vi "test.vi"() -> ()   [LabVIEW 2020, in "MSXML.lvlib"]
uses:
  Public/Type Definition/Attributes__slk_msxml.ctl
  Public/Type Definition/Attribute__slk_msxml.ctl
  MSXML.lvlib
  Public/MSXML Document/msxml document.lvclass
  Public/MSXML Node/msxml node.lvclass
panel:
  out "xml data":string
  in  "attributes":T1
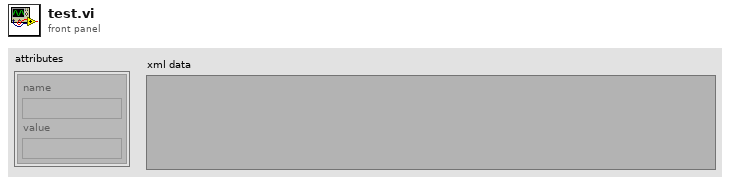
[diagram p1: front panel]
types:
  T1 = typedef "MSXML.lvlib/Attributes__slk_msxml.ctl" = T2[]
  T2 = typedef "MSXML.lvlib/Attribute__slk_msxml.ctl" = cluster{"name":string, "value":string}
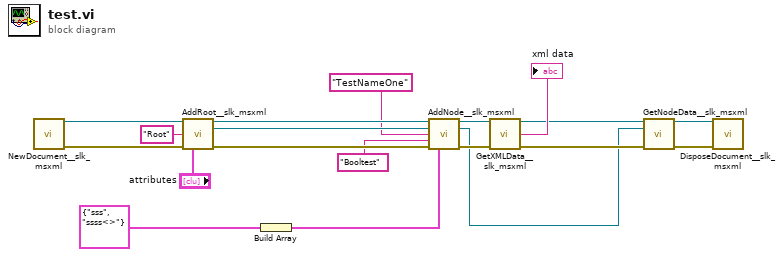
[diagram p0: block diagram]
diagram:
  n1 = call "NewDocument__slk_msxml.vi"() -> ("document out"=w19:refnum<class "msxml document.lvclass">, "error out"=w16:errorcluster)  [unwired: 14 in]
  n2 = call "AddRoot__slk_msxml.vi"("document in"=w19, "node name"="Root", "error in (no error)"=w16, "attributes"="attributes") -> ("document out"=w15:refnum<class "msxml document.lvclass">, "root node out"=w13:refnum<class "msxml node.lvclass">, "error out"=w14:errorcluster)  [unwired: 9 in]
  n3 = Build Array(T2 {"name"="sss", "value"="ssss<>"} ("attributes 2")) -> (w7:T2[])
  n4 = call "AddNode__slk_msxml.vi"("document in"=w15, "parent node in"=w13, "node name"="TestNameOne", "text"="Booltest" ("node name"), "error in (no error)"=w14, "attributes"=w7) -> ("document out"=w10:refnum<class "msxml document.lvclass">, "new node out"=w2:refnum<class "msxml node.lvclass">, "error out"=w9:errorcluster)  [unwired: 7 in]
  n5 = call "GetXMLData__slk_msxml.vi"("document in"=w10, "error in (no error)"=w9) -> ("document out"=w6:refnum<class "msxml document.lvclass">, "xml data"=→"xml data":string, "error out"=w4:errorcluster)  [unwired: 11 in]
  n6 = call "GetNodeData__slk_msxml.vi"("document in"=w6, "node in"=w2, "error in (no error)"=w4) -> ("document out"=w5:refnum<class "msxml document.lvclass">, "error out"=w3:errorcluster)  [unwired: 9 in, 2 out]
  n7 = call "DisposeDocument__slk_msxml.vi"("document in"=w5, "error in (no error)"=w3) -> ()  [unwired: 13 in, 1 out]
